vi "paging_index.vi"(9 "horizontal_scrollbar":i32, 10 "sticky_column":i32=-1, 11 "visible_columns":i32) -> (0 "post_sticky_length":i32, 1 "post_sticky_index":i32, 2 "pre_sticky_length":i32, 3 "pre_sticky_index":i32)   [LabVIEW 2015, in "lv-pagination.lvlib"]
doc: "This VI can be used to calculate the indexes of a static data set to use depending on the visible rows/columns and the values of the vertical/horizontal scrollbars."
uses:
  lv-pagination.lvlib
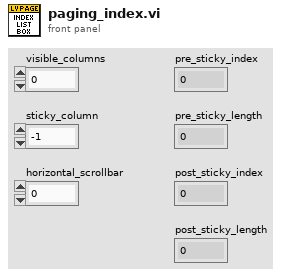
[diagram p1: front panel]
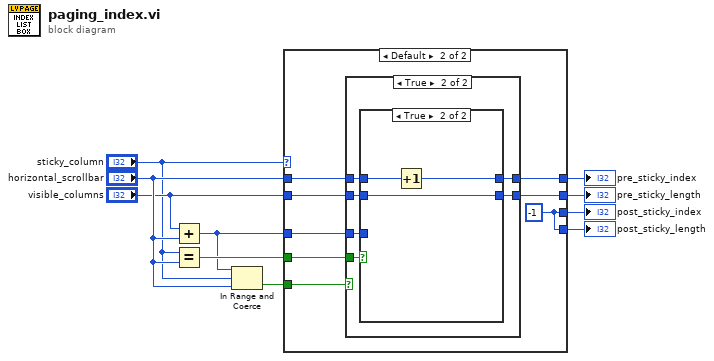
[diagram p0: block diagram]
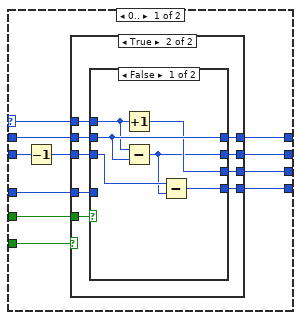
[diagram p2: hidden frame]
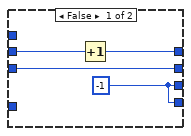
[diagram p3: hidden frame]
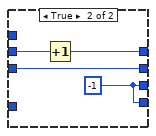
[diagram p4: hidden frame]
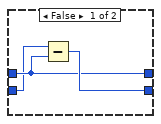
[diagram p6: hidden frame]
diagram:
  n1 = Add(x="visible_columns", y="horizontal_scrollbar") -> (x+y=w5:i32)
  n2 = Equal?(x="sticky_column", y="horizontal_scrollbar") -> (x = y?=w6:bool)
  n3 = In Range and Coerce(upper limit=w5, x="sticky_column", lower limit="horizontal_scrollbar") -> (In Range?=w4:bool)  [unwired: 1 out]
  n4 = case shown="Default" "sticky_column" {
    selector: "sticky_column" -> [w13 _]
    tunnel: [w21 w45] -> w10
    tunnel: [w20 w45] -> w9
    tunnel: [w19 w52] -> w8
    tunnel: [w18 w51] -> w7
    tunnel: w6 -> [w17 w50]
    tunnel: w5 -> [w16 w49]
    tunnel: "visible_columns" -> [w15 w48]
    tunnel: w4 -> [w14 w47]
    tunnel: "horizontal_scrollbar" -> [w12 w46]
    frame 0.. {
      n5 = Decrement(x=w15) -> (x-1=w11:i32)
      n6 = case shown="True" w14 {
        tunnel: w12 -> [w25 w34]
        tunnel: w11 -> [w24 w26]
        tunnel: [w22 w28] -> w18
        tunnel: [w24 w32] -> w19
        tunnel: [w23 w30] -> w21
        tunnel: w13 -> [_ w33]
        tunnel: [w23 w27] -> w20
        tunnel: w16 -> [_ w31]
        tunnel: w17 -> [_ w29]
        frame False {
          w23 = -1
          n7 = Increment(x=w25) -> (x+1=w22:i32)
        }
        frame True {
          n8 = case shown="False" w29 {
            tunnel: w34 -> [w39 w44]
            tunnel: w33 -> [w38 _]
            tunnel: [w35 w42] -> w32
            tunnel: w31 -> [_ _]
            tunnel: [w40 w41] -> w30
            tunnel: [w39 w43] -> w28
            tunnel: [w37 w41] -> w27
            tunnel: w26 -> [w36 w42]
            frame False {
              n9 = Increment(x=w38) -> (x+1=w37:i32)
              n10 = Subtract(x=w38, y=w39) -> (x-y=w35:i32)
              n11 = Subtract(x=w36, y=w35) -> (x-y=w40:i32)
            }
            frame True {
              w41 = -1
              n12 = Increment(x=w44) -> (x+1=w43:i32)
            }
          }
        }
      }
    }
    frame Default {
      w45 = -1
      n13 = case shown="True" w47 {
        tunnel: w46 -> [w54 w60]
        tunnel: w48 -> [w53 w55]
        tunnel: [w54 w56] -> w51
        tunnel: [w53 w59] -> w52
        tunnel: w49 -> [_ w58]
        tunnel: w50 -> [_ w57]
        frame False {
        }
        frame True {
          n14 = case shown="True" w57 {
            tunnel: w60 -> [w62 w66]
            tunnel: [w63 w64] -> w59
            tunnel: w58 -> [_ _]
            tunnel: [w62 w65] -> w56
            tunnel: w55 -> [w61 w64]
            frame False {
              n15 = Subtract(x=w61, y=w62) -> (x-y=w63:i32)
            }
            frame True {
              n16 = Increment(x=w66) -> (x+1=w65:i32)
            }
          }
        }
      }
    }
  }
  "post_sticky_length" <- w10
  "post_sticky_index" <- w9
  "pre_sticky_length" <- w8
  "pre_sticky_index" <- w7
